vi "Write Parameter File.vi"(8 "error in (no error)":errorcluster, 11 "CD Parameter Manager in":refnum<class "CD Parameter Manager.lvclass">) -> (0 "error out":errorcluster, 3 "CD Parameter Manager out":refnum<class "CD Parameter Manager.lvclass">)   [LabVIEW 2016, in "CD Parameter Manager API.lvlib" / "CD Parameter Manager.lvclass"]
uses:
  CD Parameter Manager.lvclass
  Parameter Generic File/Parameter Generic File.lvclass
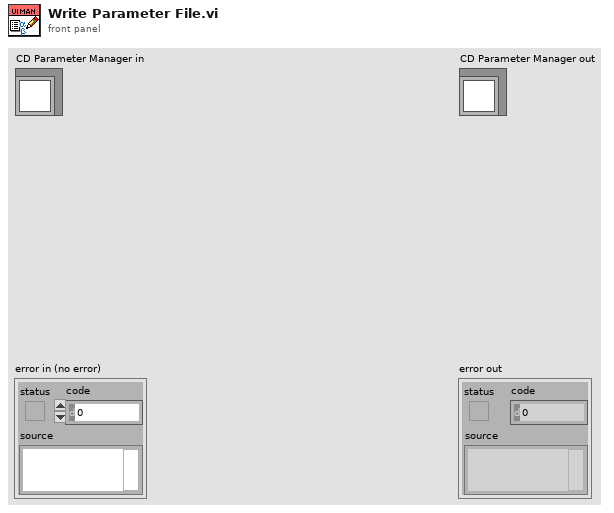
[diagram p1: front panel]
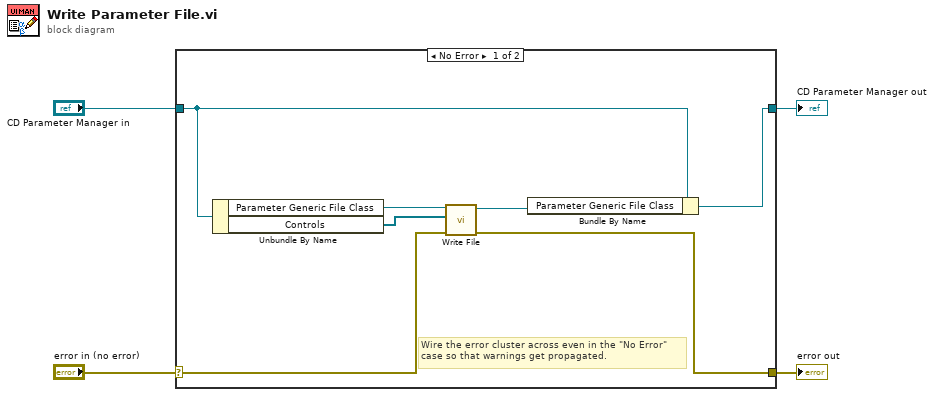
[diagram p0: block diagram]
diagram:
  n1 = case shown="No Error" "error in (no error)" {
    selector: "error in (no error)" -> [w11 w13]
    tunnel: [w10 w13] -> w3
    tunnel: [w5 w12] -> w1
    tunnel: "CD Parameter Manager in" -> [w6 w12]
    frame No Error {
      # "Wire the error cluster across even in the \"No Error\"\ncase so that warnings get propagated."
      n2 = Unbundle By Name(w6) -> ("Parameter Generic File Class"=w9:refnum<class "Parameter Generic File.lvclass">, "Controls"=w8:refnum<class "Parameter.lvclass">[])
      n3 = call-dynamic "Write File.vi"("error in (no error)"=w11, "Parameters"=w8, "Parameter Generic File in"=w9) -> ("error out"=w10:errorcluster, "Parameter Generic File out"=w7:refnum<class "Parameter Generic File.lvclass">)  [unwired: 7 in]
      n4 = Bundle By Name(cluster=w6, "Parameter Generic File Class"=w7) -> (w5:refnum<class "CD Parameter Manager.lvclass">)
    }
    frame Error {
    }
  }
  "error out" <- w3
  "CD Parameter Manager out" <- w1
